vi "HP 3458 temp monitor.vi"() -> ()   [LabVIEW 2021]
panel:
  in  "stop":bool
  out "?":cluster{dbl, dbl, dbl[]}(graph)
  in  "VISA session":refnum<visa-resource-name>
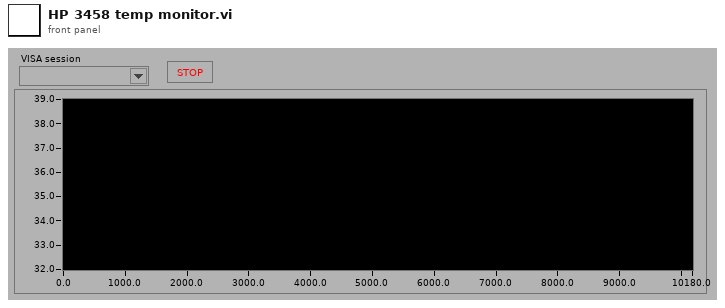
[diagram p1: front panel]
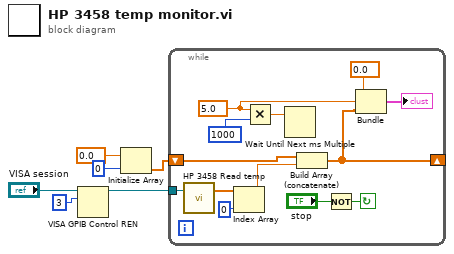
[diagram p0: block diagram]
diagram:
  n1 = VISA GPIB Control REN(10:u16 3 ("mode"), 11:"VISA session") -> (3:w1:refnum<visa-resource-name>)  [unwired: 1 in, 1 out]
  n2 = Initialize Array(0.0, 0) -> (w6:dbl[])
  n3 = while {
    tunnel: w1 -> [w13]
    shift-left: w6 -> [w16]
    shift-right: [w8] -> _
    stop <- w18 continue-if-true
    w12 = 5.0
    n4 = call "HP 3458 Read temp.vi"("VISA session"=w13) -> ("Measurement"=w17:dbl[])  [unwired: 1 in, 1 out]
    n5 = Index Array(array=w17, index=0) -> (element=w15:dbl)
    n6 = Multiply(x=w12, y=1000) -> (x*y=w11:dbl)
    n7 = Wait Until Next ms Multiple(millisecond multiple=w11) -> ()  [unwired: 1 out]
    n8 = Build Array (concatenate)(w16, w15) -> (w8:dbl[])
    n9 = Not(x="stop") -> (.not. x?=w18:bool)
    n10 = Bundle(0.0, w12, w8) -> (→"?":cluster{dbl, dbl, dbl[]})  [unwired: 1 in]
  }
